vi "new.vi"(8 "Error In":errorcluster, 10 "ref":refnum<vi>, 11 "GObject in":refnum<class "GObject.lvclass">) -> (0 "Error Out":errorcluster, 3 "GObject out":refnum<class "GObject.lvclass">)   [LabVIEW 2023, in "TLC_Scripto.lvlib" / "GObject.lvclass"]
uses:
  GObject.lvclass
  GObject.lvclass/GObject.ctl
  <userlib>/_OpenG.lib/error/error.llb/openg_error.lvlib
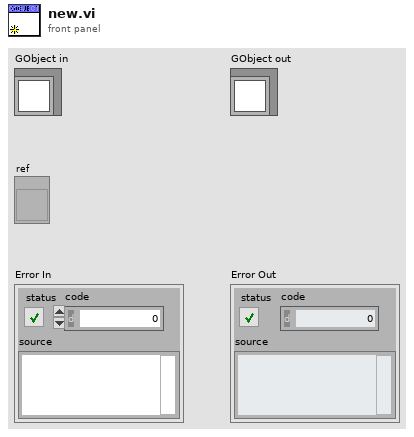
[diagram p1: front panel]
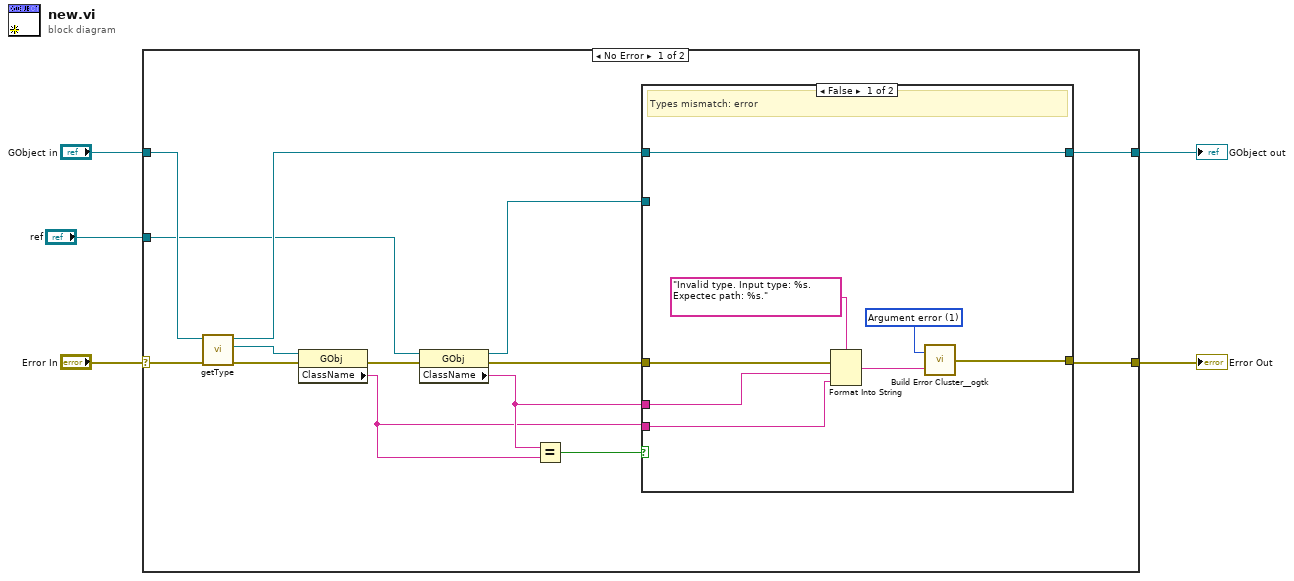
[diagram p0: block diagram]
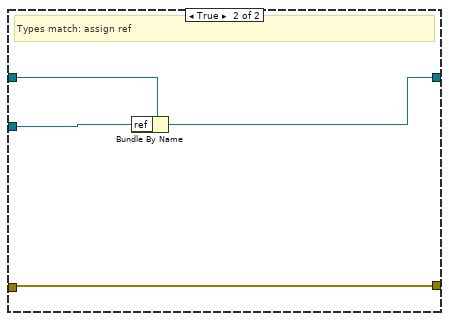
[diagram p2: hidden frame]
diagram:
  n1 = case shown="No Error" "Error In" {
    selector: "Error In" -> [w16 w32]
    tunnel: "GObject in" -> [w17 w33]
    tunnel: [w19 w33] -> w5
    tunnel: [w9 w32] -> w3
    tunnel: "ref" -> [w14 _]
    frame No Error {
      n2 = call-dynamic "getType.vi"("error in (no error)"=w16, "GObject in"=w17) -> ("error out"=w11:errorcluster, "type"=w15:refnum<vi>, "GObject out"=w18:refnum<class "GObject.lvclass">)  [unwired: 7 in]
      n3 = property class="GObj"(reference=w15, error in=w11) -> (error out=w10:errorcluster, "ClassName"=w6:string)  [unwired: 1 out]
      n4 = property class="GObj"(reference=w14, error in=w10) -> (reference out=w13:refnum<vi>, error out=w8:errorcluster, "ClassName"=w7:string)
      n5 = Equal?(x=w7, y=w6) -> (x = y?=w12:bool)
      n6 = case shown="False" w12 {
        tunnel: [w27 w31] -> w19
        tunnel: w18 -> [w27 w30]
        tunnel: w13 -> [_ w29]
        tunnel: [w23 w28] -> w9
        tunnel: w8 -> [w22 w28]
        tunnel: w7 -> [w21 _]
        tunnel: w6 -> [w20 _]
        frame False {
          w25 = 1 items=["No error", "Argument error", "Memory is full", "Out of zone", "End of file", "File already open", "Generic file I/O error", "File not found", "File permission error", "Disk is full", "Duplicate path", "Too many files open", "System feature not enabled", "Resource file not found", "Cannot add resource", "Resource not found", "Image not found", "Image memory error", "Pen does not exist", "Config type invalid", "Config token not found", "Config parse error", "Config memory error", "Bad external code format", "Bad external code offset", "External code not present", "Null window", "Destroy window error", "Null menu", "Print aborted", "Bad print record", "Print driver error", "Windows error during printing", "Memory error during printing", "Print dialog error", "Generic print error", "Invalid device refnum", "Device not found", "Device parameter error", "Device unit error", "Cannot open device", "Device call aborted", "Generic error", "Cancelled by user", "Object ID too low", "Object ID too high", "Object not in heap", "Unknown heap", "Unknown object (invalid DefProc)", "Unknown object (DefProc not in table)", "Message out of range", "Invalid (null) method", "Unknown message", "Manager call not supported", "Bad address", "Network operation in progress", "Network operation timed out", "Connection is busy", "Network attribute not supported", "Network error", "Address in use", "System out of memory", "Connection aborted", "Connection refused", "Not connected", "Already connected", "Connection closed", "Initialization error (interapplication manager)", "Bad occurrence", "Wait on unbound occurrence handler", "Occurrence queue overflow", "Datalog type conflict", "Unused", "Unrecognized type (interapplication manager)", "Memory corrupt", "Failed to make temporary DLL", "Old CIN version", "Drag socket not found", "Failed to load drop-object", "Failed to register OLE object", "Failed to release OLE object", "Format specifier type mismatch", "Unknown format specifier", "Too few format specifiers", "Too many format specifiers", "Scan failed", "Newer CIN version", "Error converting to variant", "Runtime menu error", "Password tampered", "Variant attribute not found", "Incompatible variant data type", "Event data is not available", "Event Store is not present", "Occurrence is not found", "Event Queue is not created", "Event info is not available", "Refnum passed is NULL", "Error retrieving Class GUID", "Error retrieving CoClass GUID", "Error retrieving TypeLib GUID.", "Bad built application magic bytes.", "Specific driver is different from the specific driver associated with the Logical Name.", "There is no session opened to the class driver.", "Max Error", "MAX - Error with config objects", "MAX - Error loading configuration", "MAX - Group not supported"]
          # "Types mismatch: error"
          n7 = Format Into String(format string="Invalid type. Input type: %s. Expectec path: %s.", error in=w22, w21, w20) -> (resulting string=w26:string)  [unwired: 1 in, 1 out]
          n8 = call <userlib>:"Build Error Cluster__ogtk.vi"("String to Prepend to source (\"\")"=w26, "code"=w25) -> ("error out"=w23:errorcluster)
        }
        frame True {
          # "Types match: assign ref"
          n9 = Bundle By Name(cluster=w30, "ref"=w29) -> (w31:refnum<class "GObject.lvclass">)
        }
      }
    }
    frame Error {
    }
  }
  "GObject out" <- w5
  "Error Out" <- w3
